vi "Update Series 1D U16.vi"(8 "error in (no error)":errorcluster, 9 "Image #":u32, 10 "Image Series":u16[](array[numeric]), 11 "Series Graph in":refnum<class "Series Graph.lvclass">) -> (0 "error out":errorcluster, 3 "Series Graph out":refnum<class "Series Graph.lvclass">)   [LabVIEW 2023, in "Series Graph.lvclass"]
uses:
  Series Graph.lvclass
  Base Graph/Base Graph.lvclass/Base Graph.ctl
  Base Graph/Read Sizes.vi
  Series Graph.lvclass/Series Graph.ctl
  Detail Graph/Detail Graph.lvclass
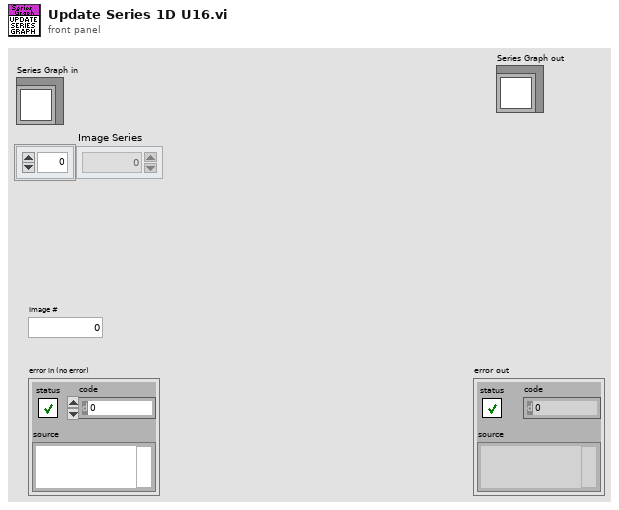
[diagram p1: front panel]
types:
  T1 = typedef "LVPointDoubleTypeDef.ctl" = cluster{"X":dbl, "Y":dbl}
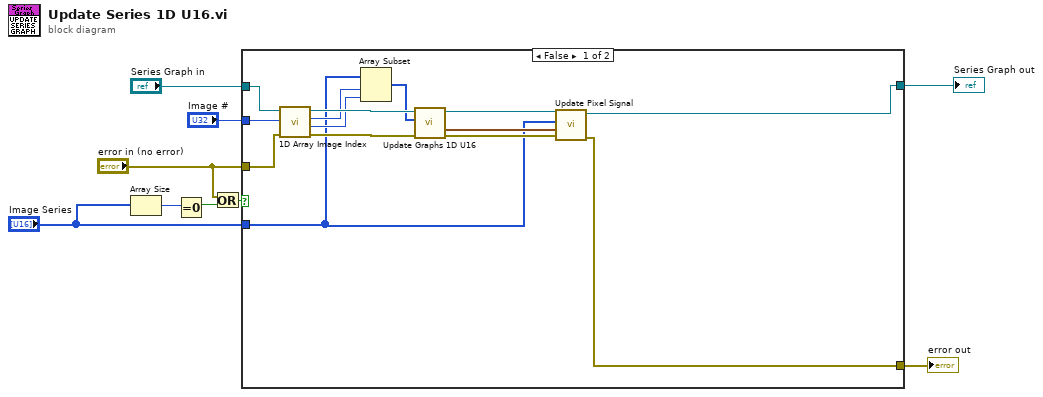
[diagram p0: block diagram]
diagram:
  n1 = Array Size(array="Image Series") -> (size(s)=w1:i32)
  n2 = Equal To 0?(x=w1) -> (x = 0?=w6:bool)
  n3 = Or(x="error in (no error)", y=w6) -> (x .or. y?=w7:bool)
  n4 = case shown="False" w7 {
    tunnel: [w12 w25] -> w9
    tunnel: [w14 w24] -> w2
    tunnel: "Image Series" -> [w10 _]
    tunnel: "Image #" -> [w22 _]
    tunnel: "error in (no error)" -> [w21 w25]
    tunnel: "Series Graph in" -> [w23 w24]
    frame False {
      n5 = call "1D Array Image Index.vi"("error in (no error)"=w21, "# Image"=w22, "Series Graph in"=w23) -> ("error out"=w18:errorcluster, "Image Length"=w16:u32, "Image Index"=w19:u32, "Series Graph out"=w20:refnum<class "Series Graph.lvclass">)  [unwired: 5 in]
      n6 = Array Subset(array=w10, index=w19, length=w16) -> (w17:u16[])
      n7 = call "Update Graphs 1D U16.vi"("error in (no error)"=w18, "image"=w17, "Detail Graph in"=w20) -> ("error out"=w13:errorcluster, "Cursor.Cursor Position"=w11:T1, "Detail Graph out"=w15:refnum<class "Series Graph.lvclass">)  [unwired: 6 in]
      n8 = call "Update Pixel Signal.vi"("error in (no error)"=w13, "Cursor.Cursor Position"=w11, "Image Series"=w10, "Series Graph in"=w15) -> ("error out"=w12:errorcluster, "Series Graph out"=w14:refnum<class "Series Graph.lvclass">)  [unwired: 6 in]
    }
    frame True {
    }
  }
  "error out" <- w9
  "Series Graph out" <- w2
